vi "Read Waveform Osciloscope.vi"(8 "error in (no error)":errorcluster, 10 "ReadWaveform":T1={"TEKTRONIX READ-WAVEFORM 2"={"Source (0: Channel 1)"=0, "Timeout (10000 ms) 2"=10000}, "EDU-X-1200A- READ-WAVEFORM"={"Bind Source Channel (2: None)"=2, "Timeout (10000 ms)"=10000, "Source Channel (0: Channel 1)"=0}} {"EDU-X-1200A- READ-WAVEFORM"."Source Channel (0: Channel 1)" items=["Channel 1"=0, "Channel 2"=1, "Channel 3"=2, "Channel 4"=3, "Waveform Memory 1"=5, "Waveform Memory 2"=6, "Serial Bus 1"=7, "Serial Bus 2"=8, "Digital Bus Low"=9, "Digital Bus High "=10, "Digital Bus 1"=11, "Digital Bus 2"=12, "External"=29, "Function 1"=32, "Function 2"=33, "Function 3"=34, "Function 4"=35, "Math 1"=36, "Math 2"=37, "Math 3"=38, "Math 4"=39, "FFT"=40, "Analog Bus"=41]; "EDU-X-1200A- READ-WAVEFORM"."Bind Source Channel (2: None)" items=["Sub Source 0", "Sub Source 1", "None"]; "TEKTRONIX READ-WAVEFORM 2"."Source (0: Channel 1)" items=["Channel 1", "Channel 2", "Channel 3", "Channel 4", "Math", "Reference A", "Reference B", "Reference C", "Reference D", "FFT"]}, 11 "EDU-X 1002A in":refnum<class "EDU-X 1002A.lvclass">) -> (0 "error out":errorcluster, 2 "Waveform Data":waveform(dbl)(graph), 3 "EDU-X 1002A out":refnum<class "EDU-X 1002A.lvclass">)   [LabVIEW 2020, in "EDU-X 1002A.lvclass"]
uses:
  EDU-X 1002A.lvclass
  TypeDefs/ReadWaveform--cluster.ctl
  EDU-X 1002A.lvclass/EDU-X 1002A.ctl
  <instrlib>/Agilent 2000 3000 X-Series/Public/Data/Read Waveforms (Single).vi
  <instrlib>/Agilent 2000 3000 X-Series/Agilent 2000 3000 X-Series.lvlib
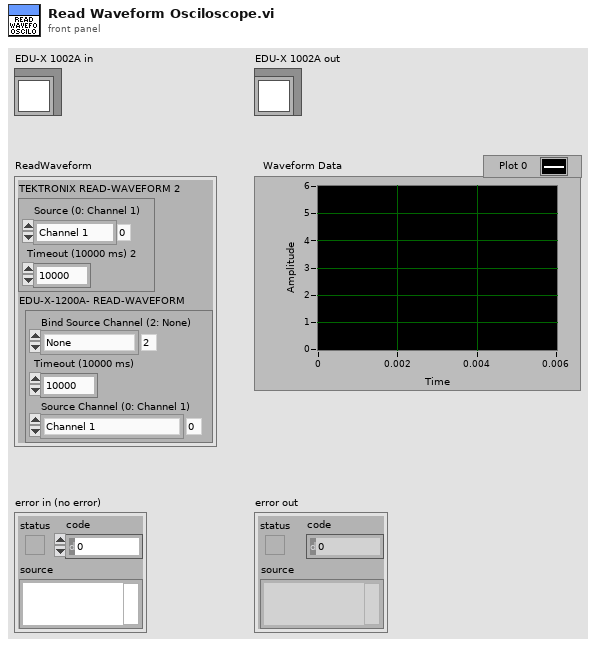
[diagram p1: front panel]
types:
  T1 = typedef "ReadWaveform--cluster.ctl" = cluster{"TEKTRONIX READ-WAVEFORM 2":cluster{"Source (0: Channel 1)":u16, "Timeout (10000 ms) 2":u32}, "EDU-X-1200A- READ-WAVEFORM":cluster{"Bind Source Channel (2: None)":i32, "Timeout (10000 ms)":u32, "Source Channel (0: Channel 1)":i32}}
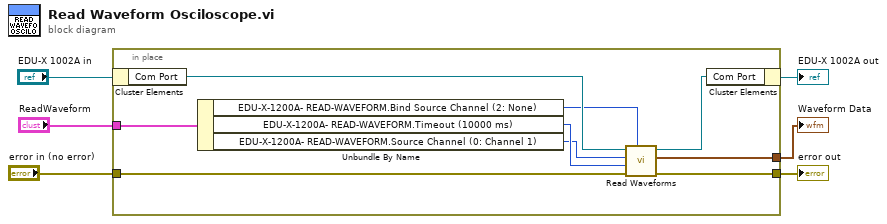
[diagram p0: block diagram]
diagram:
  n1 = in-place {
    in-place-border: "ReadWaveform" -> [w15]
    in-place-border: [w12] -> w3
    in-place-border: "error in (no error)" -> [w11]
    in-place-border: [w7] -> w1
    n2 = in-place-cluster #1("EDU-X 1002A in") -> ("Com Port"=w14:refnum<visa-resource-name>)
    n3 = Unbundle By Name(w15) -> ("EDU-X-1200A- READ-WAVEFORM.Bind Source Channel (2: None)"=w8:i32, "EDU-X-1200A- READ-WAVEFORM.Timeout (10000 ms)"=w10:u32, "EDU-X-1200A- READ-WAVEFORM.Source Channel (0: Channel 1)"=w9:i32)
    n4 = call-poly <instrlib>:"Read Waveforms.vi"("Bind Source Channel (2: None)"=w8, "error in (no error)"=w11, "Timeout (10000 ms)"=w10, "Source Channel (0: Channel 1)"=w9, "VISA resource name"=w14) -> ("error out"=w12:errorcluster, "Waveform Data"=w7:waveform(dbl), "VISA resource name out"=w13:refnum<visa-resource-name>)  [unwired: 4 in]
    n5 = in-place-cluster #1("Com Port"=w13) -> (→"EDU-X 1002A out":refnum<class "EDU-X 1002A.lvclass">)
  }
  "error out" <- w3
  "Waveform Data" <- w1
